vi "dfd_Periodic Notch Peak Filter Design.vi"(7 "filter type":T1(ring), 9 "normalized BW [rad/s]":dbl format="%.2f", 10 "Ab [dB]":dbl format="%.2f", 11 "order":i32) -> (1 "denominator":dbl[](array[numeric]) format="%.2f", 2 "numerator":dbl[](array[numeric]) format="%.2f")   [LabVIEW 2017, in "NI_DigFilter_Design.lvlib"]
uses:
  <vilib>/addons/Digital Filter Design/NI_DigFilter_Design.lvlib
  <vilib>/addons/Digital Filter Design/NI_DigFilterLicensed.lvlib
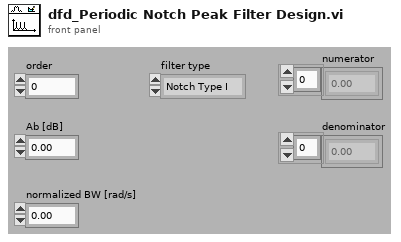
[diagram p1: front panel]
types:
  T1 = enum16{"Notch Type I", "Notch Type II", "Peak Type I", "Peak Type II"}
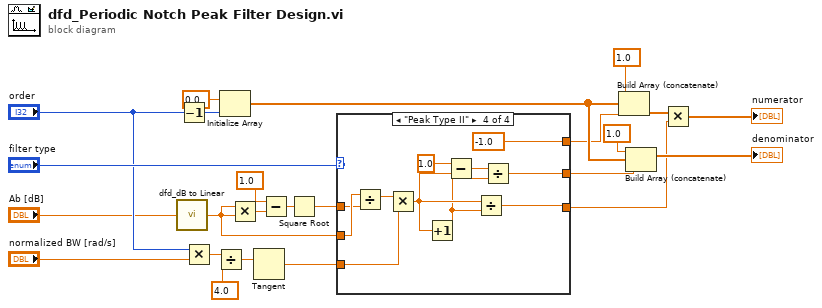
[diagram p0: block diagram]
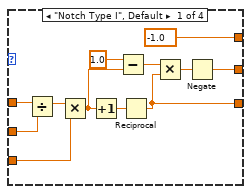
[diagram p2: hidden frame]
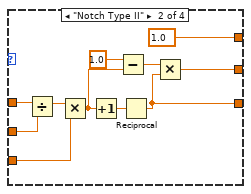
[diagram p3: hidden frame]
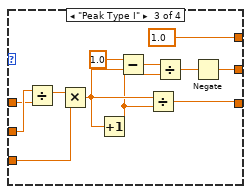
[diagram p4: hidden frame]
diagram:
  n1 = call <vilib>:"dfd_dB to Linear.vi"("dB value"="Ab [dB]") -> ("linear value"=w5:dbl)  [unwired: 1 in]
  n2 = Decrement(x="order") -> (x-1=w7:i32)
  n3 = Multiply(x="order", y="normalized BW [rad/s]") -> (x*y=w9:dbl)
  n4 = Divide(x=w9, y=4.0) -> (x/y=w13:dbl)
  n5 = Initialize Array(0.0 ("element"), w7) -> (w6:dbl[])
  n6 = Multiply(x=w5, y=w5) -> (x*y=w16:dbl)
  n7 = Tangent(1:w13) -> (0:w10:dbl)
  n8 = Subtract(x=1.0, y=w16) -> (x-y=w12:dbl)
  n9 = Square Root(x=w12) -> (sqrt(x)=w11:dbl)
  n10 = case shown="\"Peak Type II\"" "filter type" {
    tunnel: [w36 w47 w59 w70] -> w17
    tunnel: w11 -> [w35 w46 w51 w63]
    tunnel: w10 -> [w34 w45 w58 w69]
    tunnel: w5 -> [w33 w44 w52 w64]
    tunnel: [-1.0 ("element") 1.0 ("element") 1.0 ("element") -1.0 ("element")] -> w2
    tunnel: [w25 w37 w48 w60] -> w1
    frame "Notch Type I", Default {
      n11 = Divide(x=w35, y=w33) -> (x/y=w32:dbl)
      n12 = Multiply(x=w32, y=w34) -> (x*y=w28:dbl)
      n13 = Increment(x=w28) -> (x+1=w30:dbl)
      n14 = Subtract(x=1.0, y=w28) -> (x-y=w29:dbl)
      n15 = Reciprocal(x=w30) -> (1/x=w36:dbl)
      n16 = Multiply(x=w29, y=w36) -> (x*y=w26:dbl)
      n17 = Negate(x=w26) -> (-x=w25:dbl)
    }
    frame "Notch Type II" {
      n18 = Divide(x=w46, y=w44) -> (x/y=w43:dbl)
      n19 = Multiply(x=w43, y=w45) -> (x*y=w39:dbl)
      n20 = Increment(x=w39) -> (x+1=w41:dbl)
      n21 = Subtract(x=1.0, y=w39) -> (x-y=w40:dbl)
      n22 = Reciprocal(x=w41) -> (1/x=w47:dbl)
      n23 = Multiply(x=w40, y=w47) -> (x*y=w37:dbl)
    }
    frame "Peak Type I" {
      n24 = Divide(x=w52, y=w51) -> (x/y=w57:dbl)
      n25 = Multiply(x=w57, y=w58) -> (x*y=w50:dbl)
      n26 = Increment(x=w50) -> (x+1=w49:dbl)
      n27 = Subtract(x=1.0, y=w50) -> (x-y=w55:dbl)
      n28 = Divide(x=w50, y=w49) -> (x/y=w59:dbl)
      n29 = Divide(x=w55, y=w49) -> (x/y=w53:dbl)
      n30 = Negate(x=w53) -> (-x=w48:dbl)
    }
    frame "Peak Type II" {
      n31 = Divide(x=w64, y=w63) -> (x/y=w68:dbl)
      n32 = Multiply(x=w68, y=w69) -> (x*y=w62:dbl)
      n33 = Increment(x=w62) -> (x+1=w61:dbl)
      n34 = Subtract(x=1.0, y=w62) -> (x-y=w66:dbl)
      n35 = Divide(x=w62, y=w61) -> (x/y=w70:dbl)
      n36 = Divide(x=w66, y=w61) -> (x/y=w60:dbl)
    }
  }
  n37 = Build Array (concatenate)(1.0 ("element"), w6, w2) -> (w18:dbl[])
  n38 = Build Array (concatenate)(1.0 ("element"), w6, w1) -> (→"denominator":dbl[])
  n39 = Multiply(x=w18, y=w17) -> (x*y=→"numerator":dbl[])
